vi "SingleViewer.vi"   [LabVIEW 2022 SP3]
types:
  T1 = enum16{"open", "open or create", "create or replace", "create", "open (read-only)"}
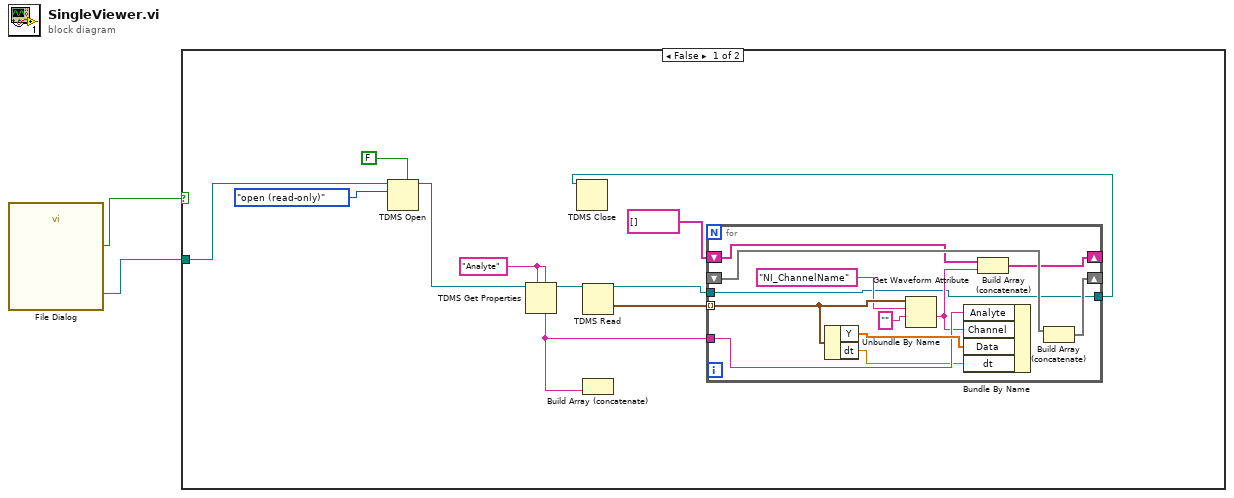
[diagram p0: block diagram]
diagram:
  n1 = call "File Dialog"() -> ("selected path"=w1:path, "cancelled"=w2:bool)  [unwired: 12 in, 2 out]
  n2 = case shown="False" w2 {
    tunnel: w1 -> [w12 _]
    frame False {
      w11 = "Analyte"
      n3 = TDMS Open(5:FALSE ("create index file? (T)"), 10:T1."open (read-only)" ("operation (0:open)"), 11:w12) -> (3:w6:refnum<k34>)  [unwired: 4 in, 1 out]
      n4 = TDMS Get Properties(5:w11, 7:w11, 11:w6) -> (3:w10:refnum<k34>, 4:w8:string)  [unwired: 3 in, 4 out]
      n5 = TDMS Read(0:w10) -> (4:w5:refnum<k34>, 10:w9:waveform(dbl)[])  [unwired: 7 in, 4 out]
      n6 = Build Array (concatenate)(w8) -> ()  [unwired: 1 in, 1 out]
      n7 = for {
        tunnel: w9 -> [w23] mode=indexing
        tunnel: w8 -> [w24]
        shift-right: [w20] -> _
        shift-left: _ -> [w19]
        shift-right: [w16] -> _
        shift-left: string[] [] -> [w17]
        tunnel: [w14] -> w4
        tunnel: w5 -> [w14]
        n8 = Unbundle By Name(w23) -> ("Y"=w25:dbl[], "dt"=w15:dbl)
        n9 = Get Waveform Attribute(5:"", 6:"NI_ChannelName" ("name"), 7:w23) -> (1:w18:string)  [unwired: 1 in, 3 out]
        n10 = Bundle By Name("Analyte"=w24, "Channel"=w18, "Data"=w25, "dt"=w15) -> ()  [unwired: 1 in, 1 out]
        n11 = Build Array (concatenate)(w17, w18) -> (w16:string[])
        n12 = Build Array (concatenate)(w19) -> (w20:void[])  [unwired: 1 in]
      }
      n13 = TDMS Close(11:w4) -> ()  [unwired: 1 in, 2 out]
    }
    frame True {
    }
  }
